vi "LSCI332 ControlSetup.vi"(6 "error in":errorcluster, 8 "Boucle(1)":u32(ring) caption="Boucle de contrôle" items=["Boucle 1", "Boucle 2"], 9 "VISA Rsrc":refnum<visa-resource-name>="GPIB0::12::INSTR" caption="Adresse du contrôlleur") -> (0 "error out":errorcluster)   [LabVIEW 2019]
doc: "Ce Vi permet la configuration des limites de contrôles ainsi que la gestion des paramètres de stabilisation. À l'ouverture, le VI lit et retourne les paramètres actuels."
uses:
  <vilib>/Utility/error.llb/DialogType.ctl
panel:
  in  "Résistance":u16=50 caption="Résistance Chauffage"
  in  "HeatUnits":u32(ring)=1 caption="Unités du chauffage" items=["Courrant"=1, "Puissance"=2]
  in  "ManOutput":dbl caption="Manual Output %" format="%#.2g"
  in  "HtrRange":u16(ring) caption="Échelle de chauffage" items=["Off", "Low (.5W)", "Med (5W)", "High (50W)"]
  in  "RampPar":cluster{"Rampe Activée":bool, "RateVal":dbl} caption="Paramètres de Rampe" {"RateVal" step=0.1}
  out "CtrlMod":bool[](array[boolean])
  in  "Réinit":bool
  in  "ZoneSetup":bool
  in  "PID":cluster{"P":dbl, "I":dbl, "D":u32}={"P"=1000.0, "I"=0.0, "D"=0} caption="Paramètres PID" {"D" max=1000 step=1; "I" min=0.0 max=1000.0 step=0.1 format="%#.1f"; "P" min=0.0 max=1000.0 step=0.1 format="%#.1f"}
  in  "SetPoint":dbl caption="Consigne"
  in  "Mode":u32(ring)=1 caption="Mode de Contrôle" items=["Manual PID"=1, "Zone"=2, "Open Loop"=3, "AutoTune PID"=4, "AutoTune PI"=5, "AutoTune P"=6]
  in  "Contrôle":bool
  in  "PowerUp":bool caption="Contrôle actif \nau démarrage"
  in  "Units":u32(ring)=1 caption="Unités du setpoint" items=["Kelvin"=1, "Celsius"=2, "Unités Capteur"=3]
  in  "Input":u32(ring) caption="Entrée de\nTempérature" items=["A", "B"]
  in  "Écrire":bool
  in  "Quit":bool
  # "Paramètres de la boucle de contrôle"
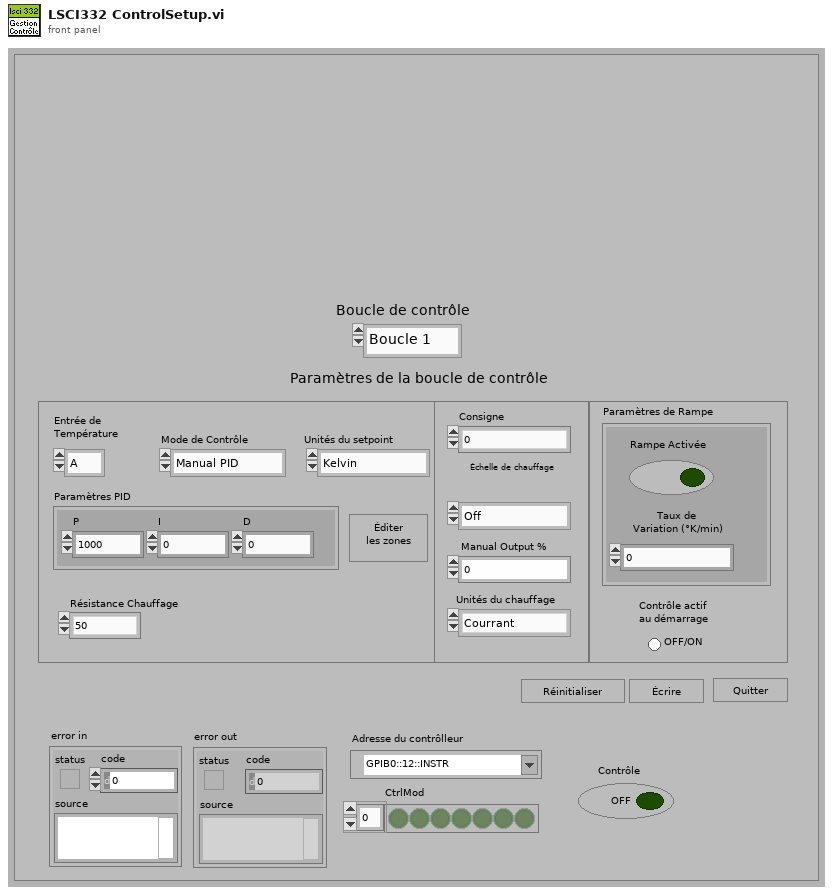
[diagram p1: front panel]
types:
  T1 = typedef "DialogType.ctl" = u16
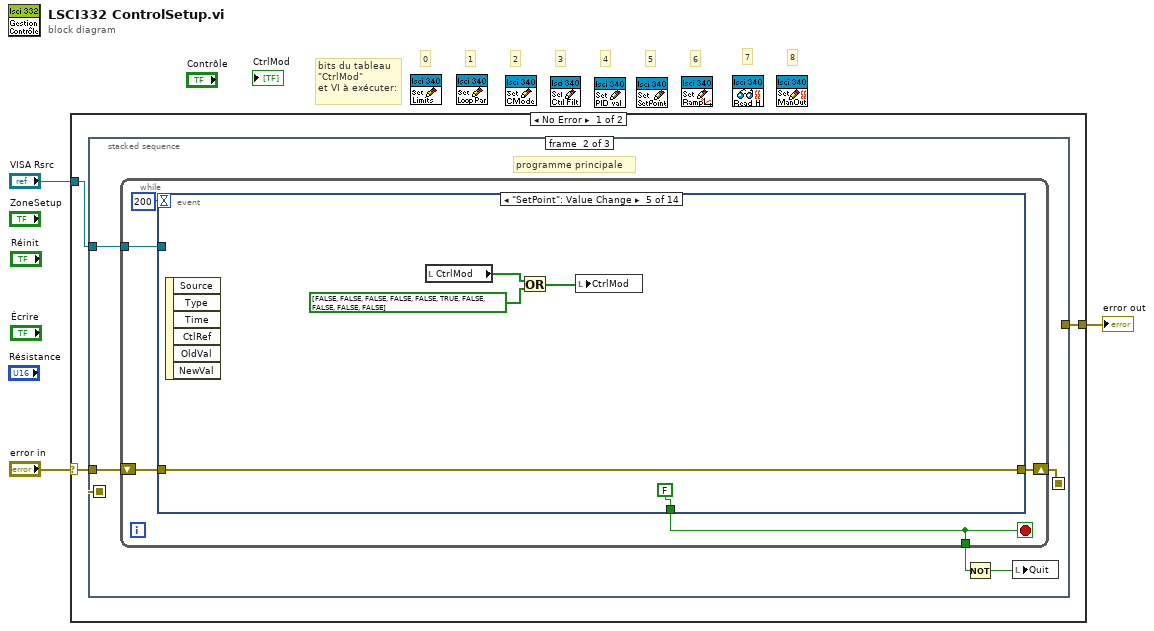
[diagram p0: block diagram]
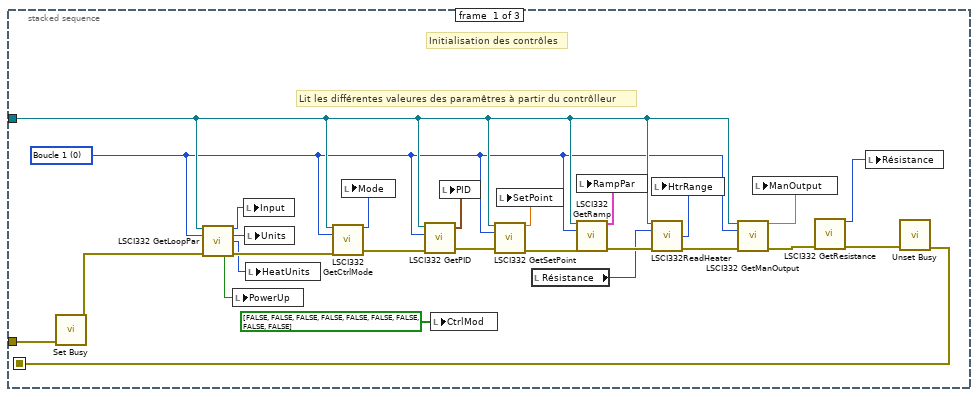
[diagram p2: hidden frame]
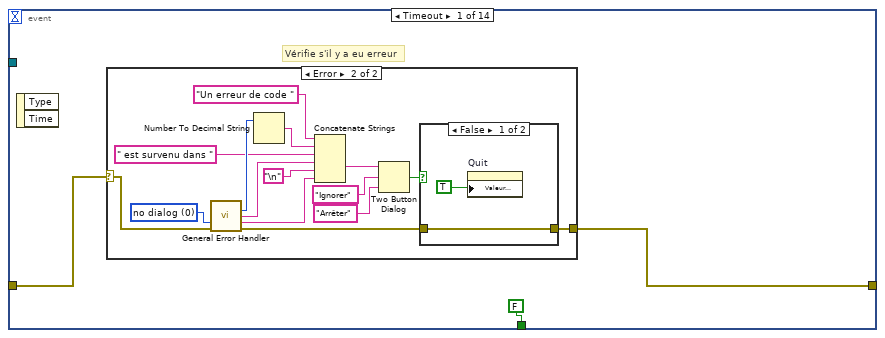
[diagram p3: hidden frame]
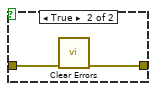
[diagram p5: hidden frame]
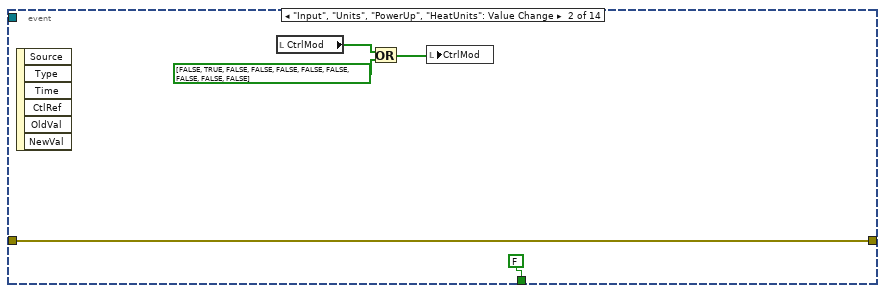
[diagram p6: hidden frame]
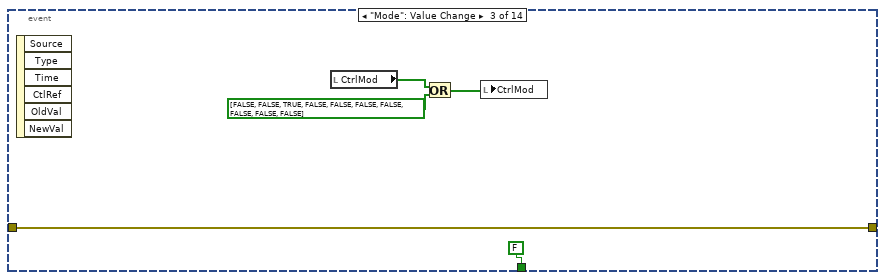
[diagram p7: hidden frame]
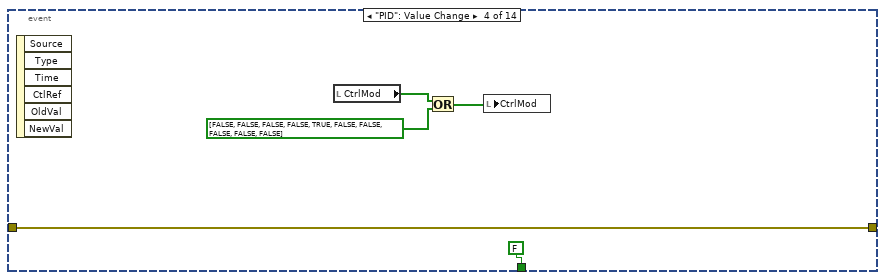
[diagram p8: hidden frame]
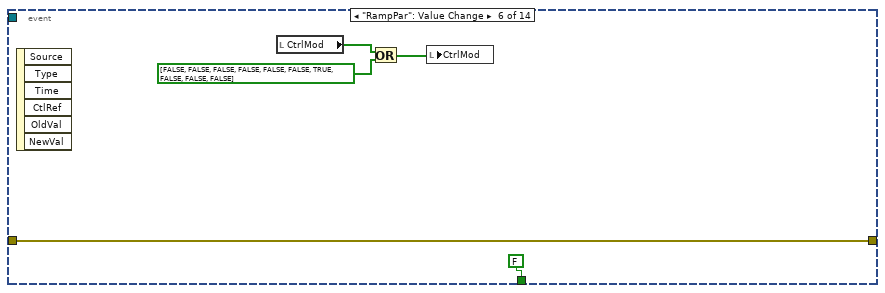
[diagram p9: hidden frame]
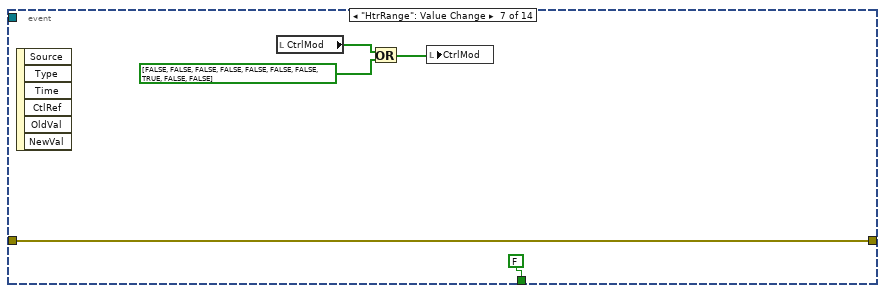
[diagram p10: hidden frame]
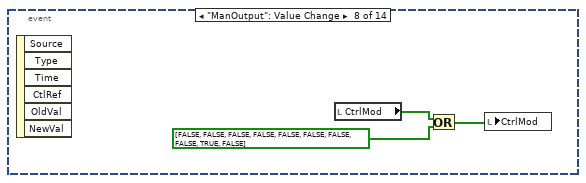
[diagram p11: hidden frame]
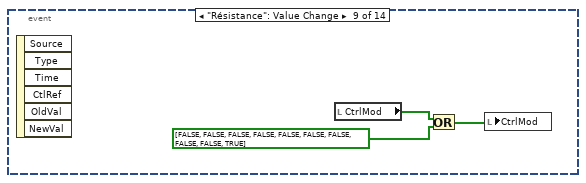
[diagram p12: hidden frame]
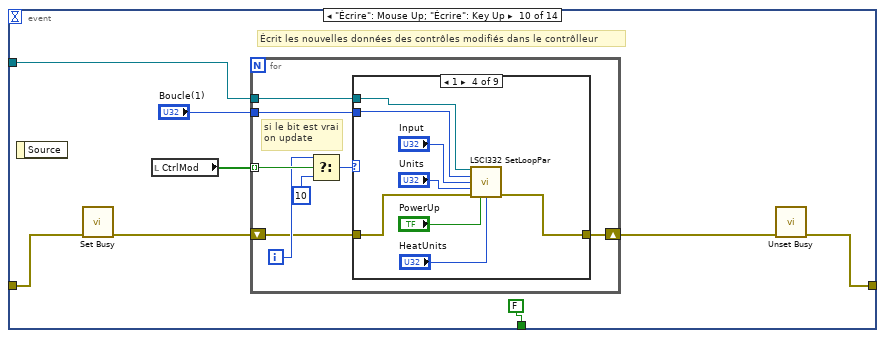
[diagram p13: hidden frame]
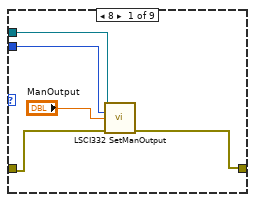
[diagram p14: hidden frame]
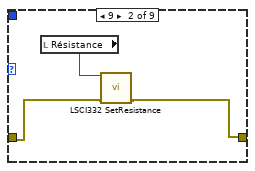
[diagram p15: hidden frame]
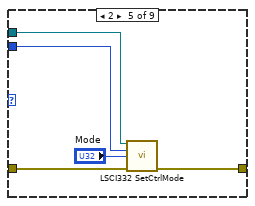
[diagram p17: hidden frame]
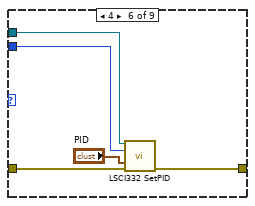
[diagram p18: hidden frame]
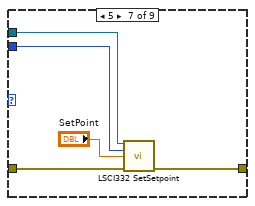
[diagram p19: hidden frame]
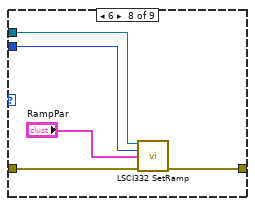
[diagram p20: hidden frame]
diagram:
  # "8"
  # "7"
  # "6"
  # "5"
  # "4"
  # "3"
  # "2"
  # "1"
  # "0"
  # "bits du tableau\n\"CtrlMod\"\net VI à exécuter:"
  n1 = case shown="No Error" "error in" {
    selector: "error in" -> [w6 w196]
    tunnel: [w4 w196] -> w2
    tunnel: "VISA Rsrc" -> [w5 _]
    frame No Error {
      n2 = stacked-sequence {
        seq-local: [w31 _ _] -> [_ w34 _]
        seq-local: [_ w33 _] -> [_ _ w195]
        tunnel: w6 -> [w32 _ _]
        tunnel: w5 -> [w15 w37 _]
        tunnel: [_ _ w194] -> w4
        frame #0 {
          w14 = u32 0 items=["Boucle 1", "Boucle 2"] ("Boucle(1)")
          # "Lit les différentes valeures des paramêtres à partir du contrôlleur"
          # "Initialisation des contrôles"
          n3 = call <vilib>:"Set Busy.vi"("error in (no error)"=w32) -> ("error out"=w12:errorcluster)  [unwired: 9 in, 1 out]
          n4 = call <userlib>:"LSCI332 GetLoopPar.vi"("VISA Rsrc"=w15, "Boucle(1)"=w14, "error in (no error)"=w12) -> ("Input"=w29:u32, "Units"=w28:u32, "HeatUnits"=w10:u32, "PowerUp"=w30:bool, "error out"=w27:errorcluster)  [unwired: 8 in]
          n5 = local write "PowerUp"(w30) -> ()
          n6 = local write "Input"(w29) -> ()
          n7 = local write "Units"(w28) -> ()
          n8 = local write "HeatUnits"(w10) -> ()
          n9 = call <userlib>:"LSCI332 GetCtrlMode.vi"("VISA Rsrc"=w15, "Boucle(1)"=w14, "error in (no error)"=w27) -> ("Mode"=w26:u32, "error out"=w11:errorcluster)  [unwired: 11 in]
          n10 = local write "Mode"(w26) -> ()
          n11 = call <userlib>:"LSCI332 GetPID.vi"("error in (no error)"=w11, "Boucle(1)"=w14, "VISA Rsrc"=w15) -> ("error out"=w24:errorcluster, "Paramètres PID"=w25:cluster{"P":dbl, "I":dbl, "D":i32})  [unwired: 6 in]
          n12 = local write "CtrlMod"(bool[] [FALSE, FALSE, FALSE, FALSE, FALSE, FALSE, FALSE, FALSE, FALSE] ("CtrlMod")) -> ()
          n13 = local write "PID"(w25) -> ()
          n14 = call <userlib>:"LSCI332 GetSetPoint.vi"("VISA Rsrc"=w15, "Boucle(1)"=w14, "error in (no error)"=w24) -> ("SetPoint"=w23:dbl, "error out"=w22:errorcluster)  [unwired: 11 in]
          n15 = local write "SetPoint"(w23) -> ()
          n16 = local read "Résistance"() -> (w9:u16)
          n17 = call <userlib>:"LSCI332 GetRamp.vi"("VISA Rsrc"=w15, "Boucle(1)"=w14, "error in (no error)"=w22) -> ("Paramètres de Rampe"=w21:cluster{"Rampe activée":bool, "RateVal":dbl}, "error out"=w20:errorcluster)  [unwired: 11 in]
          n18 = local write "RampPar"(w21) -> ()
          n19 = call <userlib>:"LSCI332ReadHeater.vi"("VISA Rsrc"=w15, "Résistance"=w9, "error in"=w20) -> ("Échelle"=w19:u16, "error out"=w17:errorcluster)  [unwired: 9 in, 2 out]
          n20 = local write "HtrRange"(w19) -> ()
          n21 = call <userlib>:"LSCI332 GetManOutput.vi"("VISA Rsrc"=w15, "Boucle(1)"=w14, "error in"=w17) -> ("ManOutput"=w16:dbl, "error out"=w13:errorcluster)  [unwired: 11 in]
          n22 = local write "ManOutput"(w16) -> ()
          n23 = call <userlib>:"LSCI332 GetResistance.vi"("error in"=w13) -> ("Résistance"=w7:u16, "error out"=w8:errorcluster)  [unwired: 13 in]
          n24 = local write "Résistance"(w7) -> ()
          n25 = call <vilib>:"Unset Busy.vi"("error in (no error)"=w8) -> ("error out"=w31:errorcluster)  [unwired: 10 in]
        }
        frame #1 {
          # "programme principale"
          n26 = while {
            shift-right: [w40] -> w33
            shift-left: w34 -> [w41]
            tunnel: w37 -> [w39]
            tunnel: [w38] -> w36
            stop <- w38 stop-if-true
            n27 = event shown="[4] \"SetPoint\": Value Change" {
              selector: _ -> [_ _ _ _ _ _ _ _ _ _ _ _ _ _]
              dyn-events: _ -> [_ _ _ _ _ _ _ _ _ _ _ _ _ _]
              timeout: 200 -> [_ _ _ _ _ _ _ _ _ _ _ _ _ _]
              tunnel: w41 -> [w45 w66 w72 w77 w82 w87 w92 _ _ w109 w161 w179 w189 w191]
              tunnel: [w44 w66 w72 w77 w82 w87 w92 _ _ w108 w160 w178 w189 w191] -> w40
              tunnel: w39 -> [_ _ _ _ _ _ _ _ _ w104 _ w170 _ _]
              tunnel: [FALSE FALSE FALSE FALSE FALSE FALSE FALSE _ _ FALSE FALSE FALSE TRUE TRUE] -> w38
              event Timeout {
                # "Vérifie s'il y a eu erreur"
                n28 = event-data() -> ()  [unwired: 1 in, 2 out]
                n29 = case shown="Error" w45 {
                  selector: w45 -> [w46 w47]
                  tunnel: [w46 w48] -> w44
                  frame No Error {
                  }
                  frame Error {
                    w58 = T1 0 items=["no dialog", "OK message", "continue or stop message", "OK message + warnings", "continue/stop + warnings"] ("type of dialog (OK msg:1)")
                    n30 = call <vilib>:"General Error Handler.vi"("type of dialog (OK msg:1)"=w58, "error in (no error)"=w47) -> ("code out"=w54:i32, "source out"=w53:string, "message"=w51:string, "error out"=w49:errorcluster)  [unwired: 9 in, 1 out]
                    n31 = Number To Decimal String(number=w54) -> (decimal integer string=w55:string)  [unwired: 1 in]
                    n32 = Concatenate Strings("Un erreur de code " ("string"), w55, " est survenu dans " ("string"), w53, "\n", w51) -> (w50:string)
                    n33 = Two Button Dialog(message=w50, 1:"Arrêter" ("F button name (\"Cancel\")"), 2:"Ignorer" ("T button name (\"OK\")")) -> (T button?=w61:bool)
                    n34 = case shown="False" w61 {
                      tunnel: w49 -> [w63 w64]
                      tunnel: [w63 w65] -> w48
                      frame False {
                        n35 = property on="Quit" class="Bool (strict)"("Valeur (Signalisation)"=TRUE ("Value (Signaling)")) -> ()  [unwired: 2 in, 2 out]
                      }
                      frame True {
                        n36 = call <vilib>:"Clear Errors.vi"("error in (no error)"=w64) -> ("error out"=w65:errorcluster)  [unwired: 5 in, 1 out]
                      }
                    }
                  }
                }
              }
              event "Input", "Units", "PowerUp", "HeatUnits": Value Change {
                n37 = event-data() -> ()  [unwired: 1 in, 6 out]
                n38 = local read "CtrlMod"() -> (w69:bool[])
                n39 = Or(x=w69, y=bool[] [FALSE, TRUE, FALSE, FALSE, FALSE, FALSE, FALSE, FALSE, FALSE, FALSE] ("Contrôles modifiés")) -> (x .or. y?=w68:bool[])
                n40 = local write "CtrlMod"(w68) -> ()
              }
              event "Mode": Value Change {
                n41 = event-data() -> ()  [unwired: 1 in, 6 out]
                n42 = local read "CtrlMod"() -> (w74:bool[])
                n43 = Or(x=w74, y=bool[] [FALSE, FALSE, TRUE, FALSE, FALSE, FALSE, FALSE, FALSE, FALSE, FALSE] ("Contrôles modifiés")) -> (x .or. y?=w73:bool[])
                n44 = local write "CtrlMod"(w73) -> ()
              }
              event "PID": Value Change {
                n45 = event-data() -> ()  [unwired: 1 in, 6 out]
                n46 = local read "CtrlMod"() -> (w80:bool[])
                n47 = Or(x=w80, y=bool[] [FALSE, FALSE, FALSE, FALSE, TRUE, FALSE, FALSE, FALSE, FALSE, FALSE]) -> (x .or. y?=w79:bool[])
                n48 = local write "CtrlMod"(w79) -> ()
              }
              event "SetPoint": Value Change {
                n49 = event-data() -> ()  [unwired: 1 in, 6 out]
                n50 = local read "CtrlMod"() -> (w84:bool[])
                n51 = Or(x=w84, y=bool[] [FALSE, FALSE, FALSE, FALSE, FALSE, TRUE, FALSE, FALSE, FALSE, FALSE] ("Contrôles modifiés")) -> (x .or. y?=w83:bool[])
                n52 = local write "CtrlMod"(w83) -> ()
              }
              event "RampPar": Value Change {
                n53 = event-data() -> ()  [unwired: 1 in, 6 out]
                n54 = local read "CtrlMod"() -> (w89:bool[])
                n55 = Or(x=w89, y=bool[] [FALSE, FALSE, FALSE, FALSE, FALSE, FALSE, TRUE, FALSE, FALSE, FALSE] ("Contrôles modifiés")) -> (x .or. y?=w88:bool[])
                n56 = local write "CtrlMod"(w88) -> ()
              }
              event "HtrRange": Value Change {
                n57 = event-data() -> ()  [unwired: 1 in, 6 out]
                n58 = local read "CtrlMod"() -> (w94:bool[])
                n59 = Or(x=w94, y=bool[] [FALSE, FALSE, FALSE, FALSE, FALSE, FALSE, FALSE, TRUE, FALSE, FALSE] ("Contrôles modifiés")) -> (x .or. y?=w93:bool[])
                n60 = local write "CtrlMod"(w93) -> ()
              }
              event "ManOutput": Value Change {
                n61 = event-data() -> ()  [unwired: 1 in, 6 out]
                n62 = local read "CtrlMod"() -> (w97:bool[])
                n63 = Or(x=w97, y=bool[] [FALSE, FALSE, FALSE, FALSE, FALSE, FALSE, FALSE, FALSE, TRUE, FALSE] ("Contrôles modifiés")) -> (x .or. y?=w96:bool[])
                n64 = local write "CtrlMod"(w96) -> ()
              }
              event "Résistance": Value Change {
                n65 = event-data() -> ()  [unwired: 1 in, 6 out]
                n66 = local read "CtrlMod"() -> (w100:bool[])
                n67 = Or(x=w100, y=bool[] [FALSE, FALSE, FALSE, FALSE, FALSE, FALSE, FALSE, FALSE, FALSE, TRUE] ("Contrôles modifiés")) -> (x .or. y?=w99:bool[])
                n68 = local write "CtrlMod"(w99) -> ()
              }
              event "Écrire": Mouse Up; "Écrire": Key Up {
                # "Écrit les nouvelles données des contrôles modifiés dans le contrôlleur"
                n69 = event-data() -> ()  [unwired: 1 in, 1 out]
                n70 = call <vilib>:"Set Busy.vi"("error in (no error)"=w109) -> ("error out"=w105:errorcluster)  [unwired: 9 in, 1 out]
                n71 = local read "CtrlMod"() -> (w106:bool[])
                n72 = for {
                  tunnel: "Boucle(1)" -> [w117]
                  tunnel: w104 -> [w116]
                  tunnel: w106 -> [w114] mode=indexing
                  shift-right: [w115] -> w103
                  shift-left: w105 -> [w110]
                  i -> [w113]
                  # "si le bit est vrai\non update"
                  n73 = Select(t=w113, s=w114, f=10) -> (s? t:f=w111:i32)
                  n74 = case shown="1" w111 {
                    tunnel: w116 -> [w122 _ _ w131 w135 w140 w145 w151 w158]
                    tunnel: w117 -> [w121 _ _ w130 w136 w141 w146 w152 _]
                    tunnel: w110 -> [w119 w125 w126 w127 w138 w143 w148 w154 w157]
                    tunnel: [w118 w124 w126 w129 w137 w142 w147 w153 w156] -> w115
                    frame 8 {
                      n75 = call <userlib>:"LSCI332 SetManOutput.vi"("VISA Rsrc"=w122, "Boucle(1)"=w121, "ManOutput"="ManOutput", "error in"=w119) -> ("error out"=w118:errorcluster)  [unwired: 11 in]
                    }
                    frame 9 {
                      n76 = local read "Résistance"() -> (w123:u16)
                      n77 = call <userlib>:"LSCI332 SetResistance.vi"("Résistance"=w123, "error in"=w125) -> ("error out"=w124:errorcluster)  [unwired: 13 in]
                    }
                    frame 10, Default {
                    }
                    frame 1 {
                      n78 = call <userlib>:"LSCI332 SetLoopPar.vi"("VISA Rsrc"=w131, "Boucle(1)"=w130, "Input"="Input", "Units"="Units", "error in (no error)"=w127, "PowerUp"="PowerUp", "HeatUnits"="HeatUnits") -> ("error out"=w129:errorcluster)  [unwired: 8 in]
                    }
                    frame 2 {
                      n79 = call <userlib>:"LSCI332 SetCtrlMode.vi"("VISA Rsrc"=w135, "Boucle(1)"=w136, "Mode"="Mode", "error in (no error)"=w138) -> ("error out"=w137:errorcluster)  [unwired: 11 in]
                    }
                    frame 4 {
                      n80 = call <userlib>:"LSCI332 SetPID.vi"("VISA Rsrc"=w140, "Boucle(1)"=w141, "Paramètres PID"="PID", "error in (no error)"=w143) -> ("error out"=w142:errorcluster)  [unwired: 11 in]
                    }
                    frame 5 {
                      n81 = call <userlib>:"LSCI332 SetSetpoint.vi"("VISA Rsrc"=w145, "Boucle(1)"=w146, "SetPoint"="SetPoint", "error in (no error)"=w148) -> ("error out"=w147:errorcluster)  [unwired: 11 in]
                    }
                    frame 6 {
                      n82 = call <userlib>:"LSCI332 SetRamp.vi"("VISA Rsrc"=w151, "Boucle(1)"=w152, "RampPar"="RampPar", "error in (no error)"=w154) -> ("error out"=w153:errorcluster)  [unwired: 11 in]
                    }
                    frame 7 {
                      n83 = call <userlib>:"LSCI332SetHeatRange.vi"("VISA Rsrc"=w158, "HtrRange"="HtrRange", "error in"=w157) -> ("error out"=w156:errorcluster)  [unwired: 12 in]
                    }
                  }
                }
                n84 = call <vilib>:"Unset Busy.vi"("error in (no error)"=w103) -> ("error out"=w108:errorcluster)  [unwired: 10 in]
              }
              event "ZoneSetup": Mouse Up; "ZoneSetup": Key Up {
                n85 = event-data() -> ()  [unwired: 1 in, 5 out]
                n86 = call <userlib>:"LSCI332 Zone Setup.vi"("error in"=w161) -> ("error out"=w160:errorcluster)  [unwired: 14 in]
              }
              event "Boucle(1)": Value Change; "Réinit": Mouse Up; "Réinit": Key Up {
                n87 = event-data() -> ()  [unwired: 1 in, 4 out]
                n88 = local read "Boucle(1)"() -> (w171:u32)
                n89 = call <vilib>:"Set Busy.vi"("error in (no error)"=w179) -> ("error out"=w167:errorcluster)  [unwired: 9 in, 1 out]
                n90 = call <userlib>:"LSCI332 GetLoopPar.vi"("VISA Rsrc"=w170, "Boucle(1)"=w171, "error in (no error)"=w167) -> ("Input"=w187:u32, "Units"=w186:u32, "HeatUnits"=w165:u32, "PowerUp"=w188:bool, "error out"=w185:errorcluster)  [unwired: 8 in]
                n91 = local write "Input"(w187) -> ()
                n92 = local write "Units"(w186) -> ()
                n93 = local write "HeatUnits"(w165) -> ()
                n94 = local write "PowerUp"(w188) -> ()
                n95 = call <userlib>:"LSCI332 GetCtrlMode.vi"("VISA Rsrc"=w170, "Boucle(1)"=w171, "error in (no error)"=w185) -> ("Mode"=w184:u32, "error out"=w166:errorcluster)  [unwired: 11 in]
                n96 = local write "Mode"(w184) -> ()
                n97 = local write "CtrlMod"(bool[] [FALSE, FALSE, FALSE, FALSE, FALSE, FALSE, FALSE, FALSE, FALSE, FALSE] ("Contrôles modifiés")) -> ()
                n98 = call <userlib>:"LSCI332 GetPID.vi"("error in (no error)"=w166, "Boucle(1)"=w171, "VISA Rsrc"=w170) -> ("error out"=w182:errorcluster, "Paramètres PID"=w183:cluster{"P":dbl, "I":dbl, "D":i32})  [unwired: 6 in]
                n99 = local write "PID"(w183) -> ()
                n100 = call <userlib>:"LSCI332 GetSetPoint.vi"("VISA Rsrc"=w170, "Boucle(1)"=w171, "error in (no error)"=w182) -> ("SetPoint"=w181:dbl, "error out"=w180:errorcluster)  [unwired: 11 in]
                n101 = local write "SetPoint"(w181) -> ()
                n102 = local read "Résistance"() -> (w164:u16)
                n103 = call <userlib>:"LSCI332 GetRamp.vi"("VISA Rsrc"=w170, "Boucle(1)"=w171, "error in (no error)"=w180) -> ("Paramètres de Rampe"=w175:cluster{"Rampe activée":bool, "RateVal":dbl}, "error out"=w173:errorcluster)  [unwired: 11 in]
                n104 = local write "RampPar"(w175) -> ()
                n105 = call <userlib>:"LSCI332ReadHeater.vi"("VISA Rsrc"=w170, "Résistance"=w164, "error in"=w173) -> ("Échelle"=w174:u16, "error out"=w169:errorcluster)  [unwired: 9 in, 2 out]
                n106 = local write "HtrRange"(w174) -> ()
                n107 = call <userlib>:"LSCI332 GetManOutput.vi"("VISA Rsrc"=w170, "Boucle(1)"=w171, "error in"=w169) -> ("ManOutput"=w172:dbl, "error out"=w168:errorcluster)  [unwired: 11 in]
                n108 = local write "ManOutput"(w172) -> ()
                n109 = call <userlib>:"LSCI332 GetResistance.vi"("error in"=w168) -> ("Résistance"=w162:u16, "error out"=w163:errorcluster)  [unwired: 13 in]
                n110 = local write "Résistance"(w162) -> ()
                n111 = call <vilib>:"Unset Busy.vi"("error in (no error)"=w163) -> ("error out"=w178:errorcluster)  [unwired: 10 in]
              }
              event "Quit": Value Change {
                # "on a appuyer sur quitter"
                n112 = event-data() -> ()  [unwired: 1 in, 6 out]
              }
              event Panel Close? {
                # "on a fermer le panneaux via le \"X\" de la barre de titre"
                n113 = event-data() -> ()  [unwired: 1 in, 4 out]
                n114 = event-data("Discard?"=TRUE) -> ()  [unwired: 1 in, 1 out]
              }
            }
          }
          n115 = Not(x=w36) -> (.not. x?=w35:bool)
          n116 = local write "Quit"(w35) -> ()
        }
        frame #2 {
          n117 = invoke class="VI" method="FP.Close"(error in=w195) -> (error out=w194:errorcluster)  [unwired: 2 in, 2 out]
        }
      }
    }
    frame Error {
    }
  }
  "error out" <- w2
